vi "Start Shutdown.vi"(8 "error in (no error)":errorcluster, 10 "stop application?":bool, 11 "controller queue":refnum<queue>) -> (0 "error out":errorcluster)   [LabVIEW 2020]
uses:
  Controller Loop/Message and Data.ctl
  Inflation Test/Parameter Class/IA Test Parameters.lvclass
  Controllers/Controller.lvclass
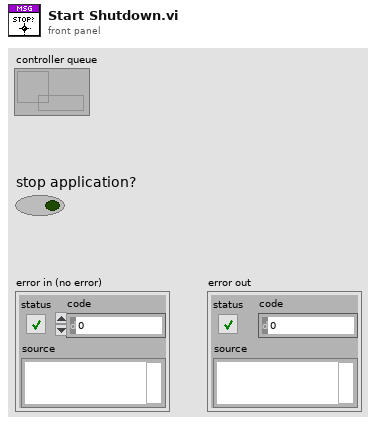
[diagram p1: front panel]
types:
  T1 = typedef "Message and Data.ctl" = cluster{"msg":string, "ia test param":refnum<class "IA Test Parameters.lvclass">, "controller type":refnum<class "Controller.lvclass">, "folder path":path, "file name":string, "file comments":string}
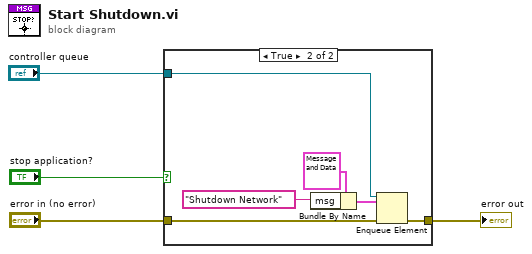
[diagram p0: block diagram]
diagram:
  n1 = case shown="True" "stop application?" {
    tunnel: [w5 w9] -> w3
    tunnel: "error in (no error)" -> [w5 w10]
    tunnel: "controller queue" -> [_ w6]
    frame False {
    }
    frame True {
      n2 = Bundle By Name(cluster=T1 {"msg"="", "ia test param"=refnum, "controller type"=refnum, "folder path"=path "", "file name"="", "file comments"=""} ("element"), "msg"="Shutdown Network") -> (w8:T1)
      n3 = Enqueue Element(queue=w6, element=w8, error in (no error)=w10) -> (error out=w9:errorcluster)  [unwired: 1 in, 2 out]
    }
  }
  "error out" <- w3
